vi "2015 HCC Cycle Stat Max.vi"(4 "2015 Cycle Stats":T1, 6 "ERD Data":T2, 8 "Error In":errorcluster, 11 "Cycle Timer":dbl format="%<%H:%M:%S>t") -> (0 "Error Out":errorcluster, 3 "2015 Cycle Stats Out":T1)   [LabVIEW 2014]
uses:
  Washer Soft Load Box/type defs/ERD_Always_Show.ctl
  Type Definitions/2015 Program/2015 Cycle Stats.ctl
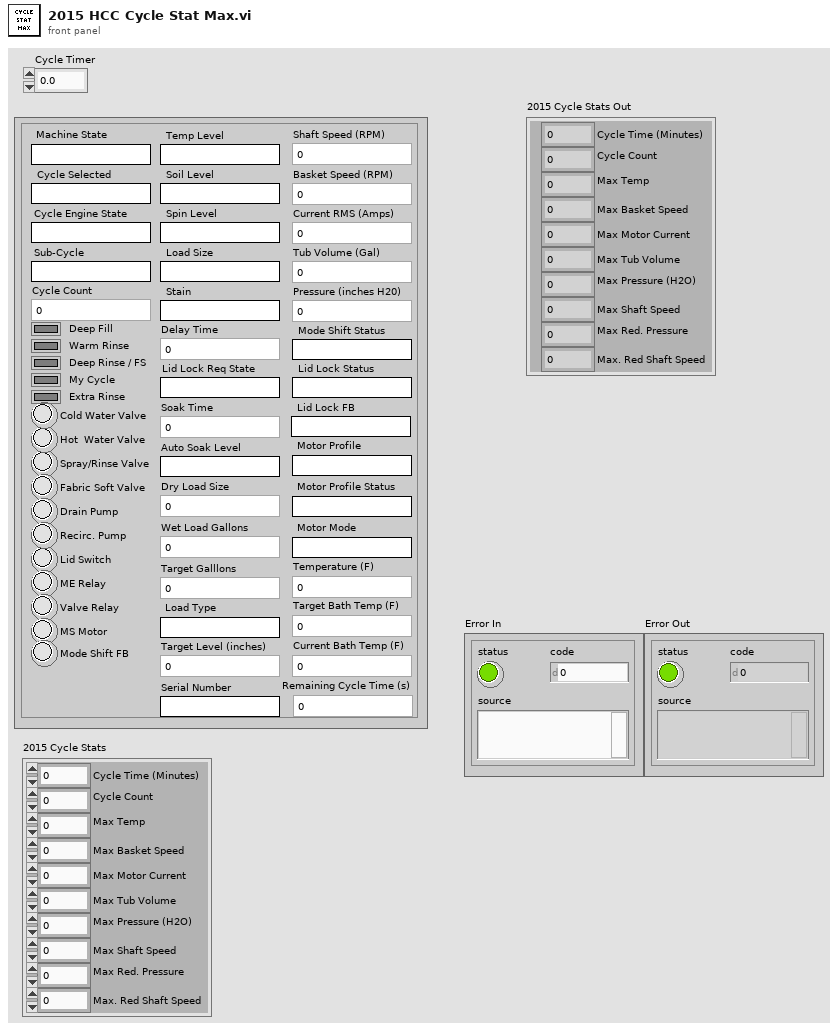
[diagram p1: front panel]
types:
  T1 = typedef "2015 Cycle Stats.ctl" = cluster{"Cycle Time (Minutes)":dbl, "Max Temp":dbl, "Max Basket Speed":dbl, "Max Motor Current":dbl, "Max Tub Volume":dbl, "Max Pressure (H2O)":dbl, "Cycle Count":dbl, "Max Shaft Speed ":dbl, "Max Red. Pressure":dbl, "Max. Red Shaft Speed":dbl}
  T2 = typedef "ERD_Always_Show.ctl" = cluster{"Basket Speed (RPM)":u16, "Machine State":string, "Tub Volume (Gal)":dbl, "Pressure (inches H20)":dbl, "Lid Switch ":bool, "Current RMS (Amps)":dbl, "Cycle Selected":string, "Lid Lock Status":string, "Mode Shift Status":string, "Spray/Rinse Valve":bool, "Fabric Soft Valve":bool, "Drain Pump":bool, "Recirc. Pump":bool, "Cycle Engine State":string, "Hot  Water Valve":bool, "Cold Water Valve":bool, "Motor Profile":string, "Motor Profile Status":string, "Motor Mode":string, "ME Relay":bool, "Cycle Count":u32, "Deep Rinse / FS":bool, "My Cycle":bool, "Soil Level":string, "Spin Level":string, "Stain":string, "Temp Level":string, "Load Size":string, "Delay Time":u16, "Soak Time":u16, "Deep Fill":bool, "Warm Rinse":bool, "Auto Soak Level":string, "Extra Rinse":bool, "Wet Load Gallons":dbl, "Target Galllons":dbl, "Sub-Cycle":string, "Load Type":string, "Target Level (inches)":u32, "Valve Relay":bool, "Dry Load Size":dbl, "Shaft Speed (RPM) ":u16, "MS Motor":bool, "Mode Shift FB":bool, "Target Bath Temp (F)":dbl, "Temperature (F)":dbl, "Current Bath Temp (F)":dbl, "Lid Lock FB":string, "Lid Lock Req State":string, "Remaining Cycle Time (s)":dbl, "Serial Number":string}
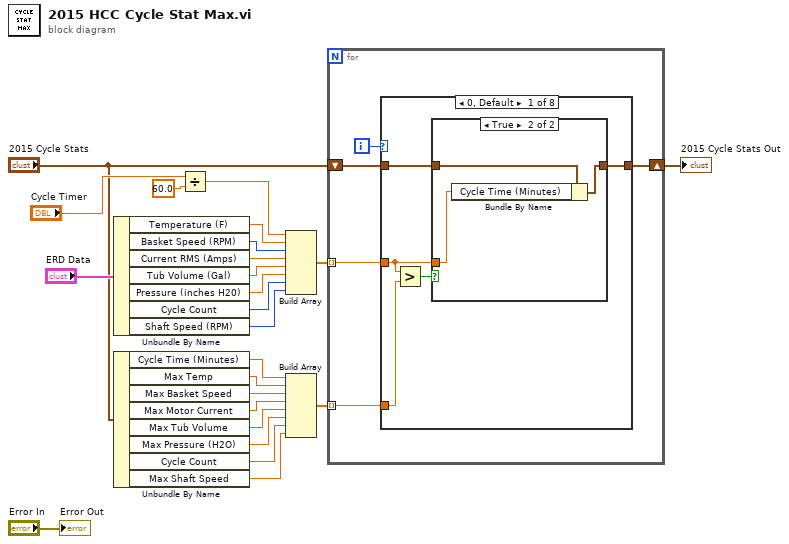
[diagram p0: block diagram]
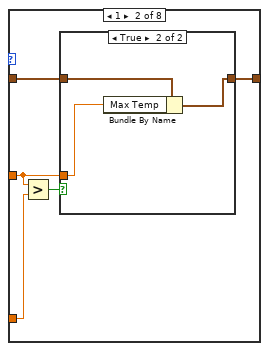
[diagram p3: hidden frame]
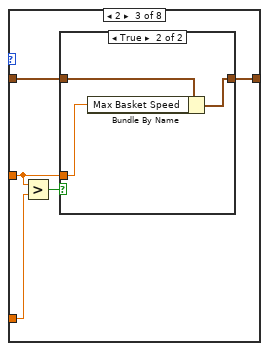
[diagram p5: hidden frame]
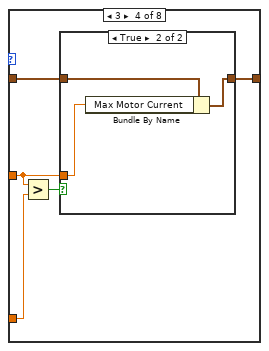
[diagram p7: hidden frame]
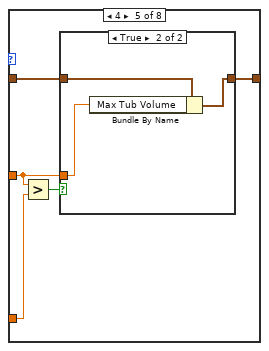
[diagram p9: hidden frame]
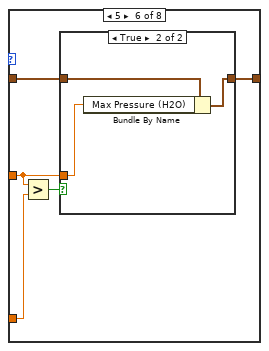
[diagram p11: hidden frame]
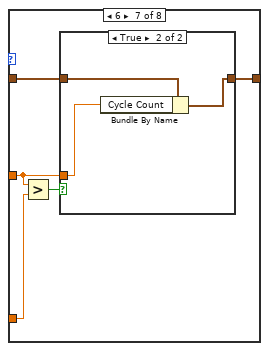
[diagram p13: hidden frame]
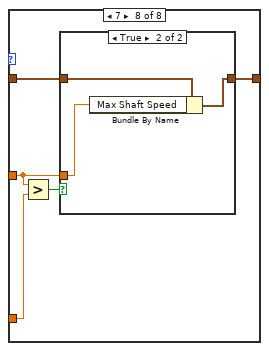
[diagram p15: hidden frame]
diagram:
  n1 = Unbundle By Name("ERD Data") -> ("Temperature (F)"=w12:dbl, "Basket Speed (RPM)"=w11:u16, "Current RMS (Amps)"=w10:dbl, "Tub Volume (Gal)"=w9:dbl, "Pressure (inches H20)"=w8:dbl, "Cycle Count"=w7:u32, "Shaft Speed (RPM)"=w6:u16)
  n2 = Unbundle By Name("2015 Cycle Stats") -> ("Cycle Time (Minutes)"=w23:dbl, "Max Temp"=w22:dbl, "Max Basket Speed"=w21:dbl, "Max Motor Current"=w20:dbl, "Max Tub Volume"=w19:dbl, "Max Pressure (H2O)"=w18:dbl, "Cycle Count"=w17:dbl, "Max Shaft Speed"=w16:dbl)
  n3 = Divide(x="Cycle Timer", y=60.0) -> (x/y=w13:dbl)
  n4 = Build Array(w13, w12, w11, w10, w9, w8, w7, w6) -> (w3:dbl[])
  n5 = Build Array(w23, w22, w21, w20, w19, w18, w17, w16) -> (w2:dbl[])
  n6 = for {
    shift-right: [w27] -> w5
    shift-left: "2015 Cycle Stats" -> [w28]
    tunnel: w3 -> [w26] mode=indexing
    tunnel: w2 -> [w25] mode=indexing
    i -> [w29]
    n7 = case shown="0, Default" w29 {
      tunnel: w28 -> [w34 w43 w52 w61 w70 w79 w88 w97]
      tunnel: [w33 w42 w51 w60 w69 w78 w87 w96] -> w27
      tunnel: w26 -> [w30 w40 w48 w58 w67 w76 w85 w94]
      tunnel: w25 -> [w32 w41 w49 w59 w68 w77 w86 w95]
      frame 0, Default {
        n8 = Greater?(x=w30, y=w32) -> (0:w31:bool)
        n9 = case shown="True" w31 {
          tunnel: w34 -> [w35 w38]
          tunnel: [w35 w37] -> w33
          tunnel: w30 -> [_ w36]
          frame False {
          }
          frame True {
            n10 = Bundle By Name(cluster=w38, "Cycle Time (Minutes)"=w36) -> (w37:T1)
          }
        }
      }
      frame 1 {
        n11 = Greater?(x=w40, y=w41) -> (0:w39:bool)
        n12 = case shown="True" w39 {
          tunnel: w43 -> [w44 w47]
          tunnel: [w44 w46] -> w42
          tunnel: w40 -> [_ w45]
          frame False {
          }
          frame True {
            n13 = Bundle By Name(cluster=w47, "Max Temp"=w45) -> (w46:T1)
          }
        }
      }
      frame 2 {
        n14 = Greater?(x=w48, y=w49) -> (0:w50:bool)
        n15 = case shown="True" w50 {
          tunnel: w52 -> [w53 w56]
          tunnel: [w53 w55] -> w51
          tunnel: w48 -> [_ w54]
          frame False {
          }
          frame True {
            n16 = Bundle By Name(cluster=w56, "Max Basket Speed"=w54) -> (w55:T1)
          }
        }
      }
      frame 3 {
        n17 = Greater?(x=w58, y=w59) -> (0:w57:bool)
        n18 = case shown="True" w57 {
          tunnel: w61 -> [w62 w65]
          tunnel: [w62 w64] -> w60
          tunnel: w58 -> [_ w63]
          frame False {
          }
          frame True {
            n19 = Bundle By Name(cluster=w65, "Max Motor Current"=w63) -> (w64:T1)
          }
        }
      }
      frame 4 {
        n20 = Greater?(x=w67, y=w68) -> (0:w66:bool)
        n21 = case shown="True" w66 {
          tunnel: w70 -> [w71 w74]
          tunnel: [w71 w73] -> w69
          tunnel: w67 -> [_ w72]
          frame False {
          }
          frame True {
            n22 = Bundle By Name(cluster=w74, "Max Tub Volume"=w72) -> (w73:T1)
          }
        }
      }
      frame 5 {
        n23 = Greater?(x=w76, y=w77) -> (0:w75:bool)
        n24 = case shown="True" w75 {
          tunnel: w79 -> [w80 w83]
          tunnel: [w80 w82] -> w78
          tunnel: w76 -> [_ w81]
          frame False {
          }
          frame True {
            n25 = Bundle By Name(cluster=w83, "Max Pressure (H2O)"=w81) -> (w82:T1)
          }
        }
      }
      frame 6 {
        n26 = Greater?(x=w85, y=w86) -> (0:w84:bool)
        n27 = case shown="True" w84 {
          tunnel: w88 -> [w89 w92]
          tunnel: [w89 w91] -> w87
          tunnel: w85 -> [_ w90]
          frame False {
          }
          frame True {
            n28 = Bundle By Name(cluster=w92, "Cycle Count"=w90) -> (w91:T1)
          }
        }
      }
      frame 7 {
        n29 = Greater?(x=w94, y=w95) -> (0:w93:bool)
        n30 = case shown="True" w93 {
          tunnel: w97 -> [w98 w101]
          tunnel: [w98 w100] -> w96
          tunnel: w94 -> [_ w99]
          frame False {
          }
          frame True {
            n31 = Bundle By Name(cluster=w101, "Max Shaft Speed"=w99) -> (w100:T1)
          }
        }
      }
    }
  }
  "2015 Cycle Stats Out" <- w5
  "Error Out" <- "Error In"
